vi "data file saver.vi"(8 "error in (no error)":errorcluster, 9 "Header String":string, 10 "default data file name":string="fred", 11 "reference file path in":path) -> (0 "error out":errorcluster, 3 "data file path out":path)   [LabVIEW 2014]
doc: "This VI creates the data file and places the header text. The data spreadsheet is added later.\n\nPaul K Dixon\nPhysics 350\nCSUSB Physics"
panel:
  # "Data file starter"
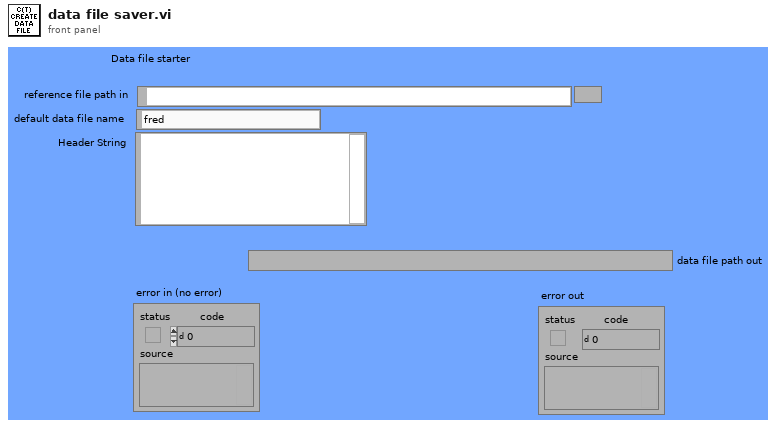
[diagram p1: front panel]
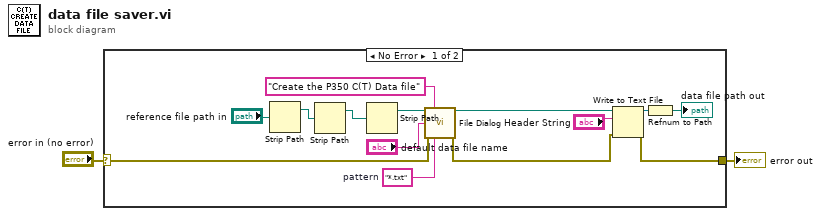
[diagram p0: block diagram]
diagram:
  n1 = case shown="No Error" "error in (no error)" {
    selector: "error in (no error)" -> [w3 w17]
    tunnel: [w11 w17] -> w1
    frame No Error {
      w7 = "*.txt"  # pattern
      n2 = Strip Path(path="reference file path in") -> (stripped path=w15:path)  [unwired: 1 out]
      n3 = Strip Path(path=w15) -> (stripped path=w10:path)  [unwired: 1 out]
      n4 = Strip Path(path=w10) -> (stripped path=w6:path)  [unwired: 1 out]
      n5 = call "File Dialog"("start path"=w6, "prompt"="Create the P350 C(T) Data file", "default name"="default data file name", "error in"=w3, "pattern (all files)"=w7) -> ("selected path"=w5:path, "error out"=w4:errorcluster)  [unwired: 7 in, 2 out]
      n6 = Write to Text File(file (use dialog)=w5, text="Header String", error in=w4) -> (refnum out=w13:refnum<file>, error out=w11:errorcluster)  [unwired: 2 out]
      n7 = Refnum to Path(1:w13) -> (0:→"data file path out":path)
    }
    frame Error {
    }
  }
  "error out" <- w1
